vi "3.2.1-VectorNav Str2Array.vi"(11 "String":string) -> (3 "Array":dbl[](array[numeric]))   [LabVIEW 2010]
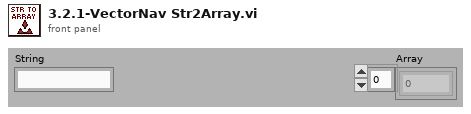
[diagram p1: front panel]
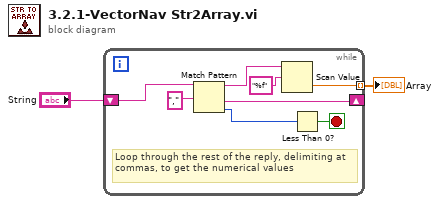
[diagram p0: block diagram]
diagram:
  n1 = while {
    shift-right: [w8] -> _
    shift-left: "String" -> [w10]
    tunnel: [w3] -> w1 mode=indexing
    stop <- w6 stop-if-true
    # "Loop through the rest of the reply, delimiting at commas, to get the numerical values"
    n2 = Match Pattern(string=w10, regular expression=",") -> (before substring=w4:string, after substring=w8:string, offset past match=w7:i32)  [unwired: 2 out]
    n3 = Scan Value(string=w4, format string="%f") -> (value=w3:dbl)  [unwired: 1 in, 1 out]
    n4 = Less Than 0?(x=w7) -> (x < 0?=w6:bool)
  }
  "Array" <- w1
